vi "Multichannel Recording0.7.vi"() -> ()   [LabVIEW 2014]
uses:
  Multichannel Record/Enum State Typedef.ctl
  Consumer Data_ Consumer Event Com.ctl
  Multichannel Record/Data Producer States.ctl
  <vilib>/_DAQmxBase/Internals/DAQmxBase Read (Analog 2D DBL NChan NSamp).vi
  <vilib>/_DAQmxBase/Internals/DAQmxBase Create Channel (AI-Voltage-Basic).vi
  <vilib>/_DAQmxBase/Internals/DAQmxBase Timing (Sample Clock).vi
panel:
  out "Progress (% / 100)":dbl(slide) scale=0.0..1.0
  in  "Display Size":T1(ring)
  out "Total Iterations Needed":dbl
  out "Read Data":i32
  out "Data Producer State":T2=enum."Default"
  out "Data Consumer State":T3=enum."Default"
  in  "Open Button":bool
  in  "Tab Control":T4(tab)
  in  "Amplifier Channel 0":T5 {"Amplifier Model" items=["Select a Model", "AM 1700", "BMA 200"]}
  out "Channel 0 Chart":waveform(dbl)(graph)
  in  "User Data Channel 0":T6
  in  "Use Channel 0":bool caption="In Use?"
  out "Channel 1 Chart":waveform(dbl)(graph)
  in  "User Data Channel 1":T6
  in  "Amplifier Channel 1":T5 {"Amplifier Model" items=["Select a Model", "AM 1700", "BMA 200"]}
  in  "Use Channel 1":bool caption="In Use?"
  out "Channel 2 Chart":waveform(dbl)(graph)
  in  "User Data Channel 2":T6
  in  "Amplifier Channel 2":T5 {"Amplifier Model" items=["Select a Model", "AM 1700", "BMA 200"]}
  in  "Use Channel 2":bool caption="In Use?"
  out "Channel 3 Chart":waveform(dbl)(graph)
  in  "User Data Channel 3":T6
  in  "Amplifier Channel 3":T5 {"Amplifier Model" items=["Select a Model", "AM 1700", "BMA 200"]}
  in  "Use Channel 3":bool caption="In Use?"
  out "Overview Chart":waveform(dbl)[](graph)
  in  "Stop Preview":bool
  in  "OK Button":bool
  out "Event State":T7
  in  "Clear Display":bool
  in  "Preview Button":bool
  out "Iterations Recorded":i32
  in  "Recording Time (seconds)":dbl
  in  "Sample Rate":i64=1000
  in  "Stop Button":bool
  out "Start Time hr/min":string
  out "Date mm/dd/yy":string
  in  "Exit Button":bool
  in  "Record Button":bool
  # "MSU EFISH Lab Multi-Channel Electronic Pulse Recorder"
  # "Must enter numbers into here before you start"
  # "Blue for On\nOrange for Off"
  # "DC"
  # "AC"
  # "Blue for AC and Orange for DC"
  # "Blue for On\nOrange for Off"
  # "DC"
  # "AC"
  # "Blue for AC and Orange for DC"
  # "Blue for On\nOrange for Off"
  # "DC"
  # "AC"
  # "Blue for AC and Orange for DC"
  # "Blue for On\nOrange for Off"
  # "DC"
  # "AC"
  # "Blue for AC and Orange for DC"
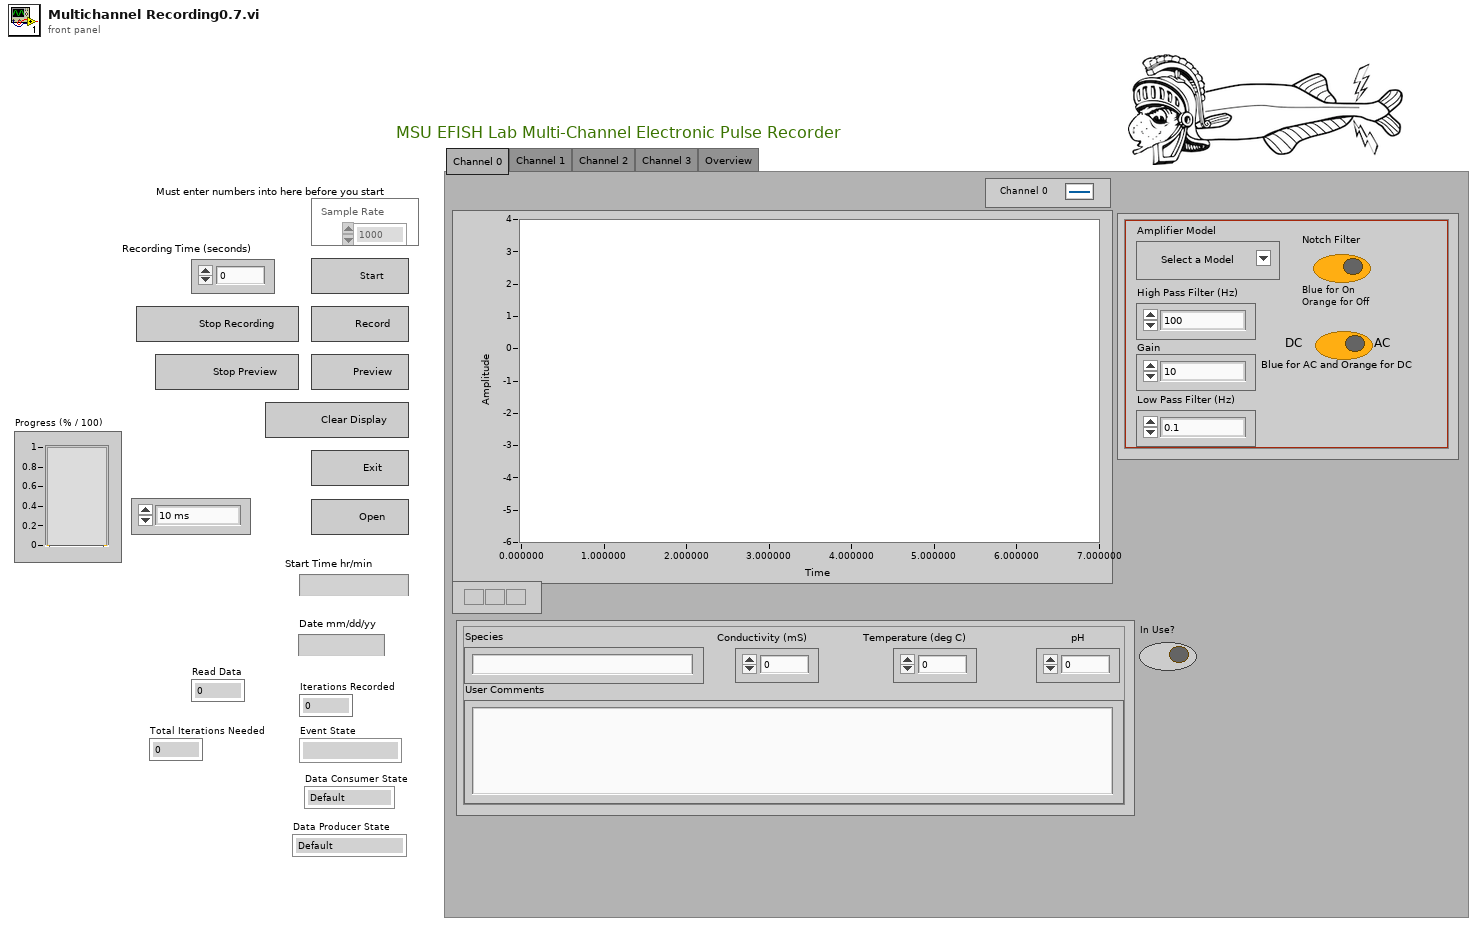
[diagram p1: front panel]
types:
  T1 = enum16{"10 ms", "100 ms", "1 Second", "10 sec", "30 sec"}
  T2 = typedef "Data Producer States.ctl" = enum16{"Read Data", "Set Sample Clock", "Default", "Exit", "Preview"}
  T3 = typedef "Consumer Data_ Consumer Event Com.ctl" = enum16{"Recording", "Create File", "Clear Memory", "Default", "End File", "Exit", "Set Sample Clock", "Preview"}
  T4 = enum32{"Channel 0", "Channel 1", "Channel 2", "Channel 3", "Overview"}
  T5 = cluster{"Low Pass Filter (Hz)":enum16{"0.1", "1", "3", "10", "30", "100", "300"}, "Gain ":enum16{"10", "20", "50", "100", "200", "500", "1000", "2k", "5k", "10k", "20k", "50k"}, "High Pass Filter (Hz)":enum16{"100", "500", "1000", "3000", "5000", "10,000", "20,000", "30,000", "50,000"}, "Notch Filter":bool, "Amplifier Model":u16, "AC/DC Switch":bool}
  T6 = cluster{"pH":dbl, "Conductivity (mS)":dbl, "Temperature (deg C)":dbl, "User Comments":string, "Species":string}
  T7 = typedef "Enum State Typedef.ctl" = enum16{"", "Open FIle", "Beginning State", "Set the Sample Clock", "Prepreview Handling", "Clear Display", "Preview Data", "Stop", "Exit", "Record", "Create File"}
  T8 = enum8{"Enabled", "Disabled", "Disabled and Grayed Out"}
  T9 = enum16{"Recording", "Create File", "Clear Memory", "Default"}
  T10 = cluster{"Refnum out":refnum<k34>, "Refnum out":refnum<k34>, "Refnum out":refnum<k34>, "Refnum out":refnum<k34>}
  T11 = cluster{"Use Channel 0":bool, "Use Channel 1":bool, "Use Channel 2":bool, "Use Channel 3":bool}
  T12 = cluster{"tdms file out":refnum<k34>, "tdms file out":refnum<k34>, "tdms file out":refnum<k34>, "tdms file out":refnum<k34>}
  T13 = cluster{"Channel 0 Chart":refnum<vi>, "Channel 1 Chart":refnum<vi>, "Channel 2 Chart":refnum<vi>, "Channel 3 Chart":refnum<vi>, "Overview Chart":refnum<vi>}
  T14 = cluster{"Waveform":waveform(dbl), "Waveform":waveform(dbl), "Waveform":waveform(dbl), "Waveform":waveform(dbl), waveform(dbl)[]}
  T15 = enum16{"Read Data", "Set Sample Clock", "Default", "Exit"}
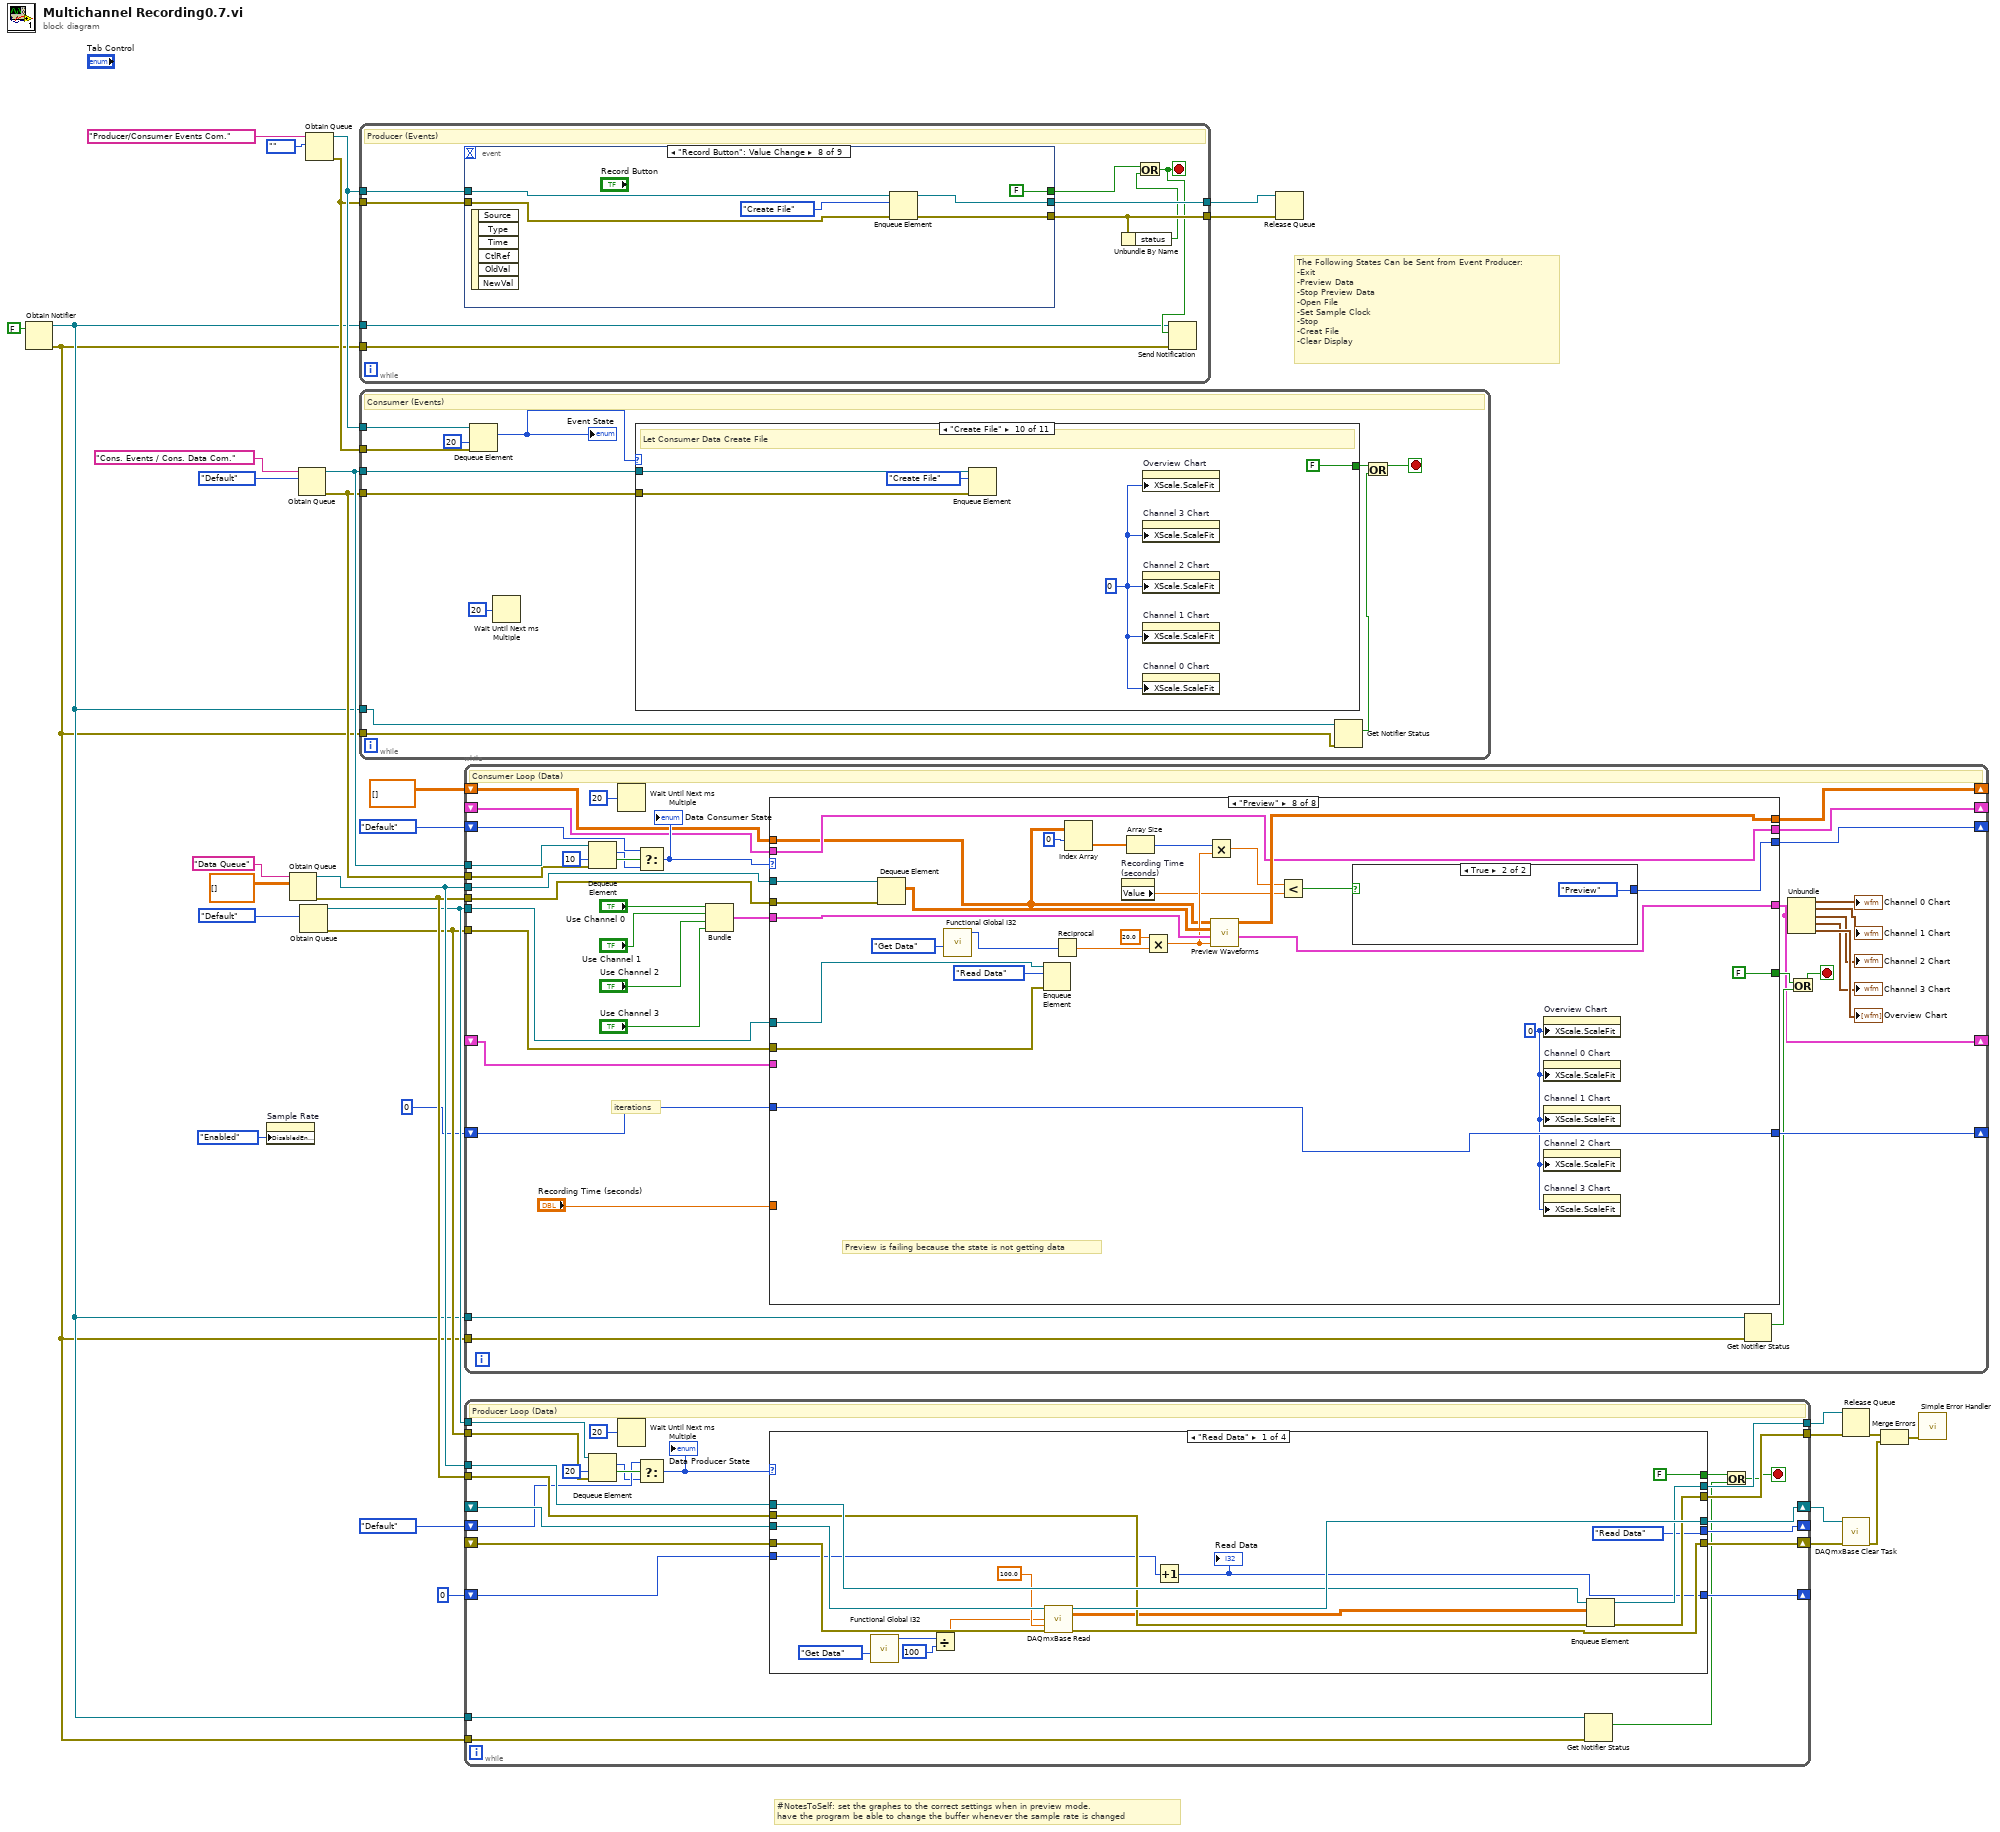
[diagram p0: block diagram]
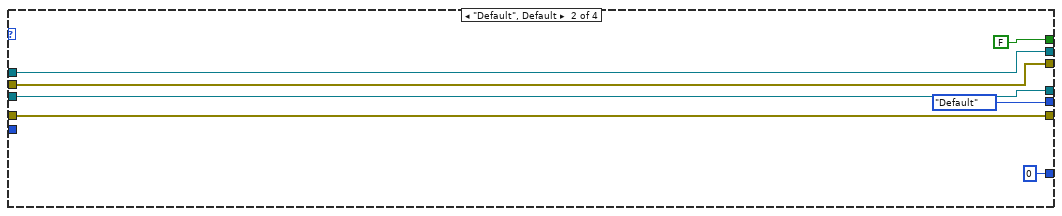
[diagram p2: hidden frame]
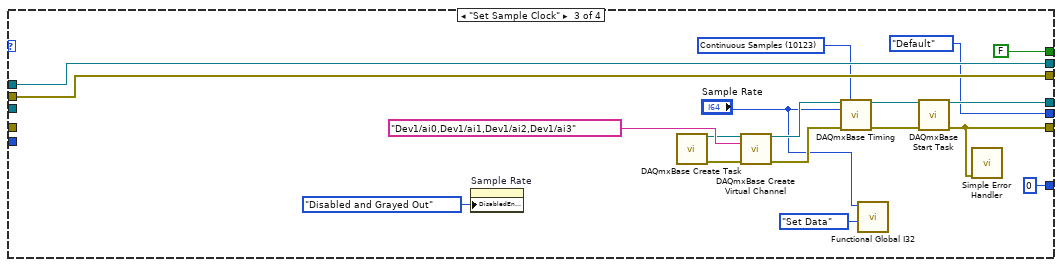
[diagram p3: hidden frame]
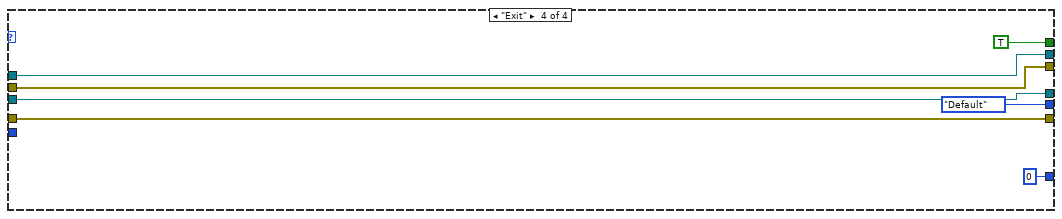
[diagram p4: hidden frame]
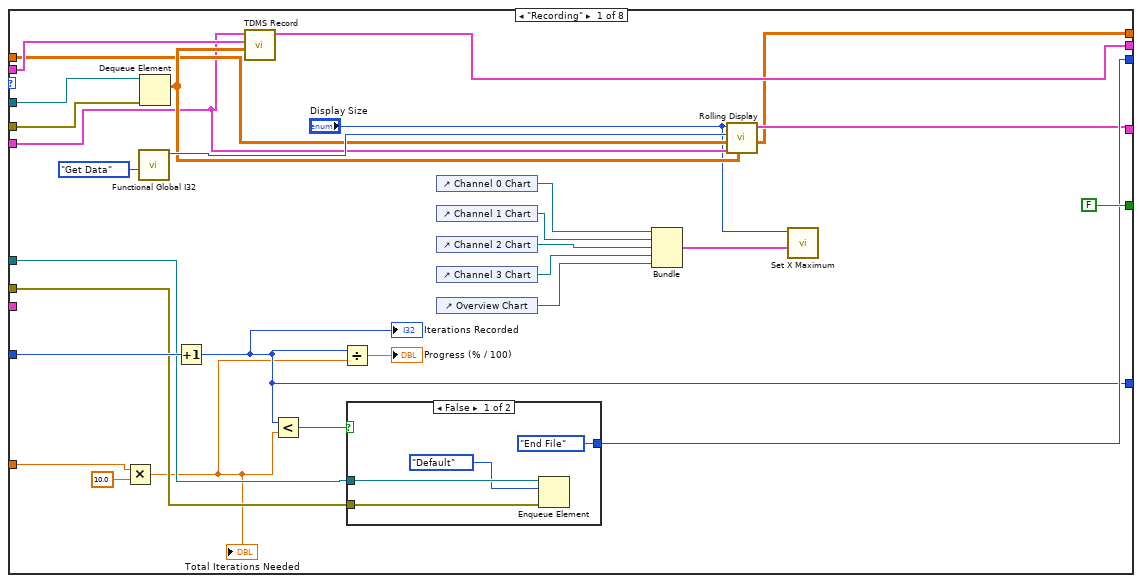
[diagram p5: hidden frame]
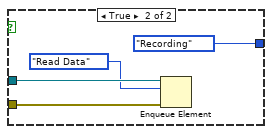
[diagram p6: hidden frame]
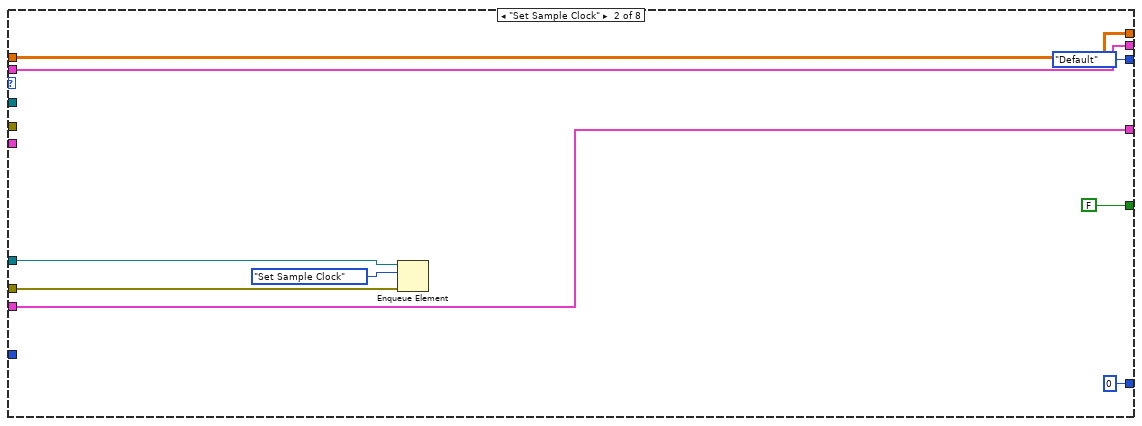
[diagram p7: hidden frame]
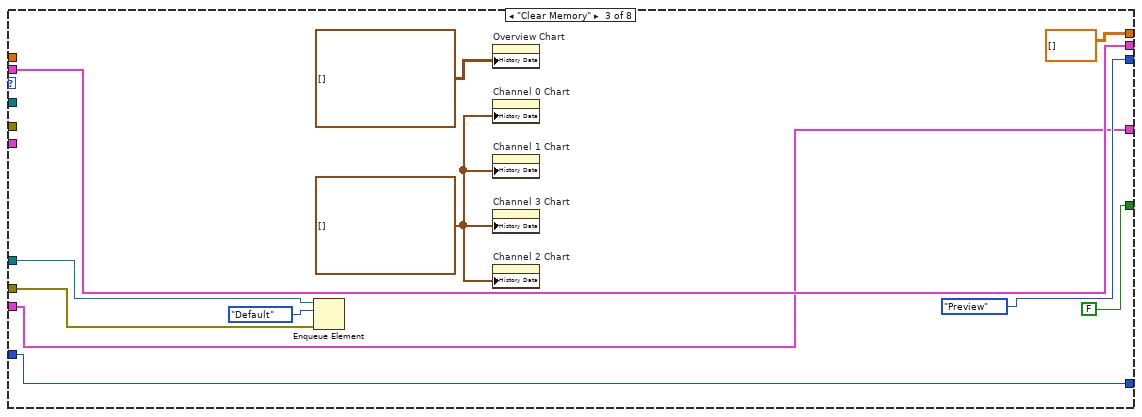
[diagram p8: hidden frame]
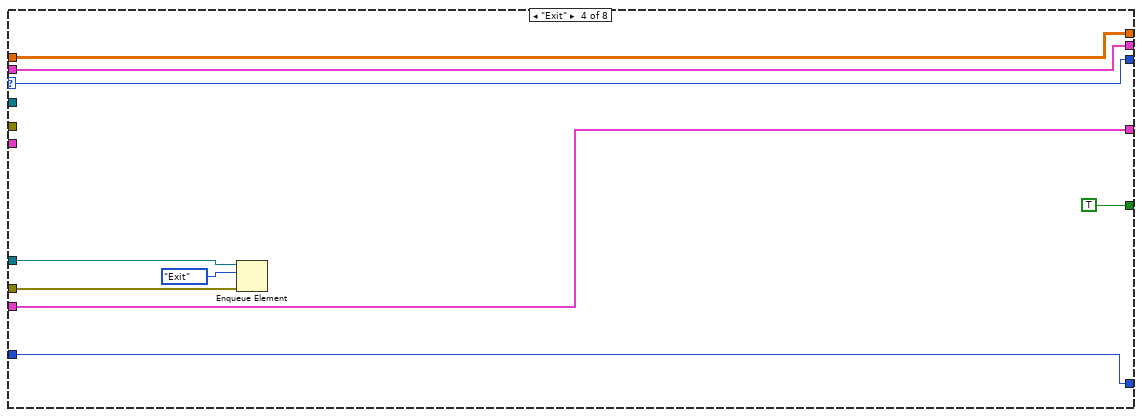
[diagram p9: hidden frame]
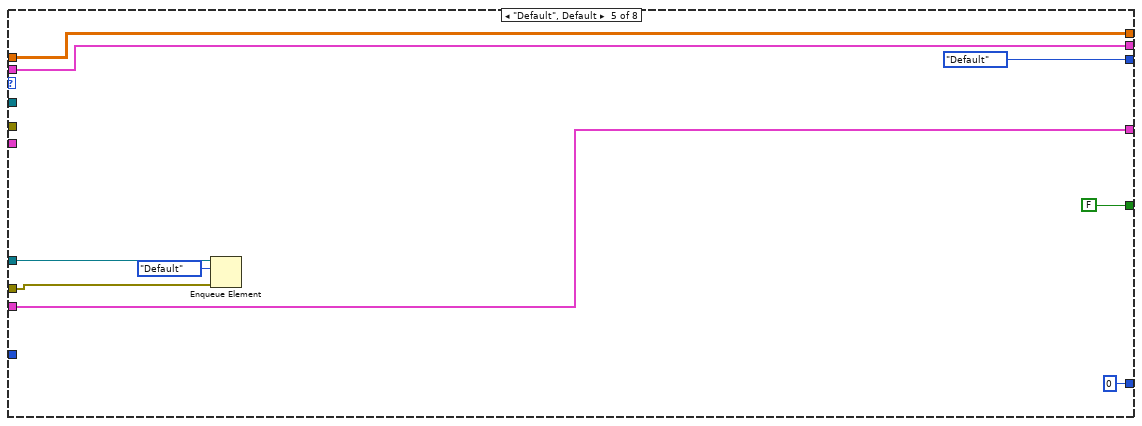
[diagram p10: hidden frame]
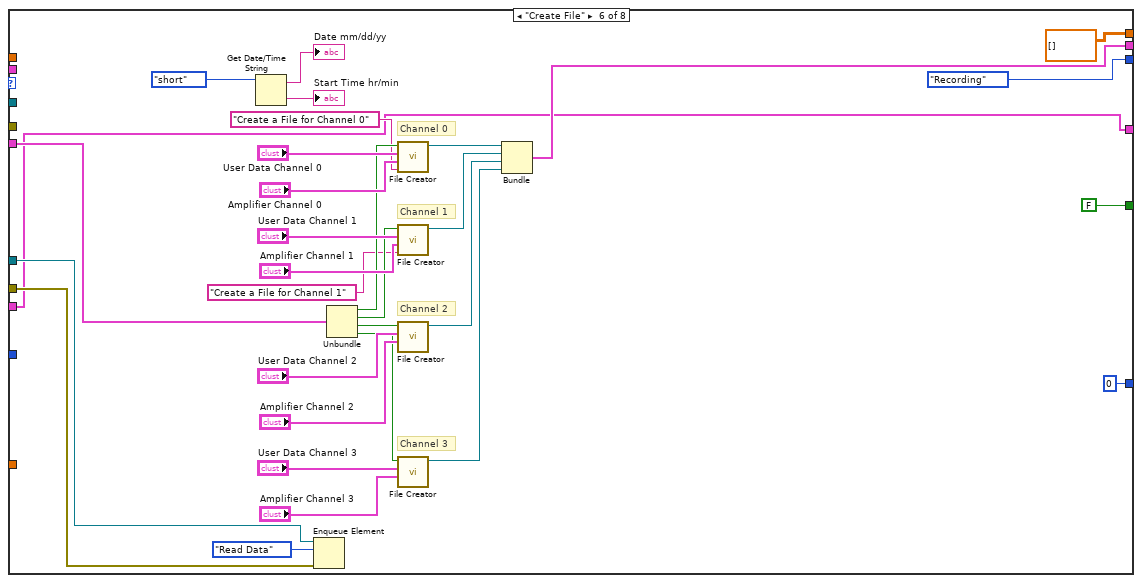
[diagram p11: hidden frame]
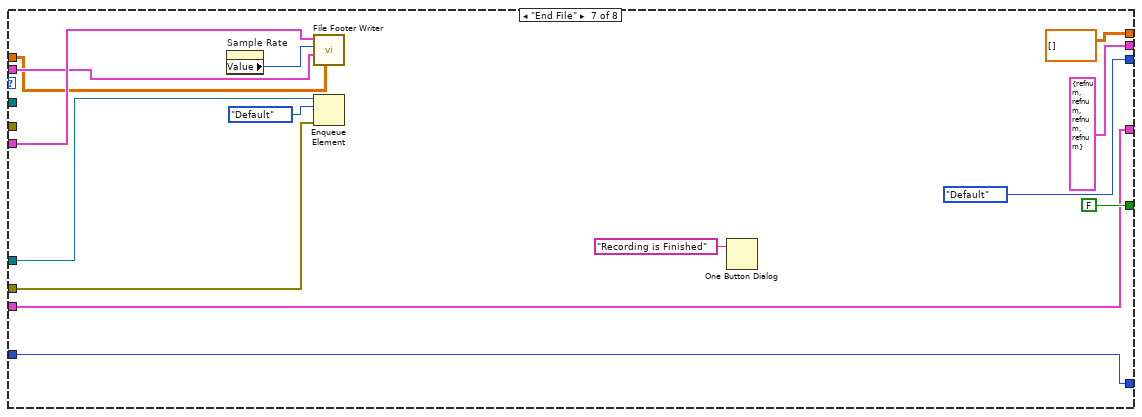
[diagram p12: hidden frame]
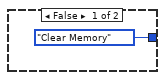
[diagram p13: hidden frame]
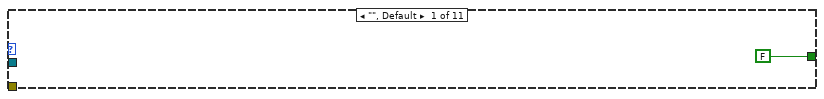
[diagram p14: hidden frame]
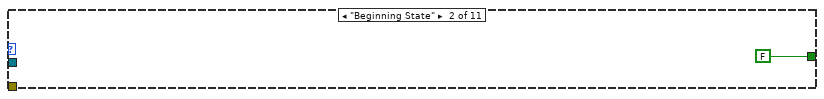
[diagram p15: hidden frame]
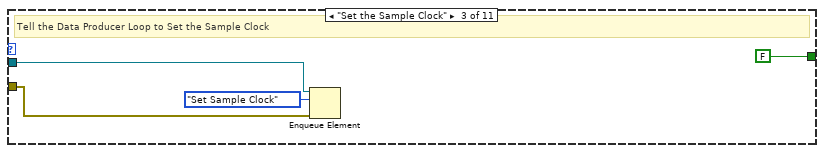
[diagram p16: hidden frame]
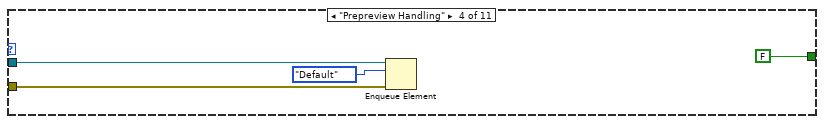
[diagram p17: hidden frame]
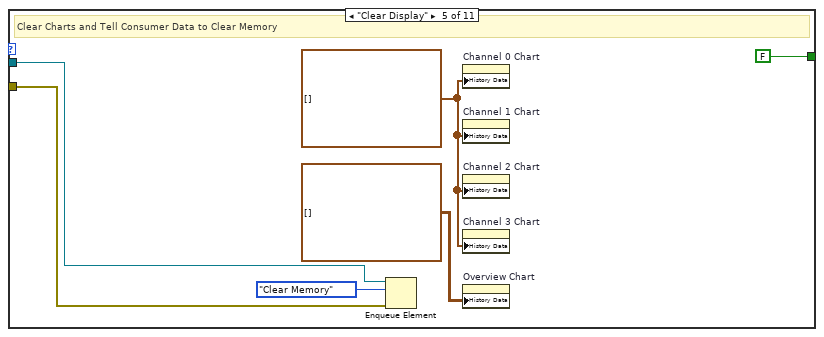
[diagram p18: hidden frame]
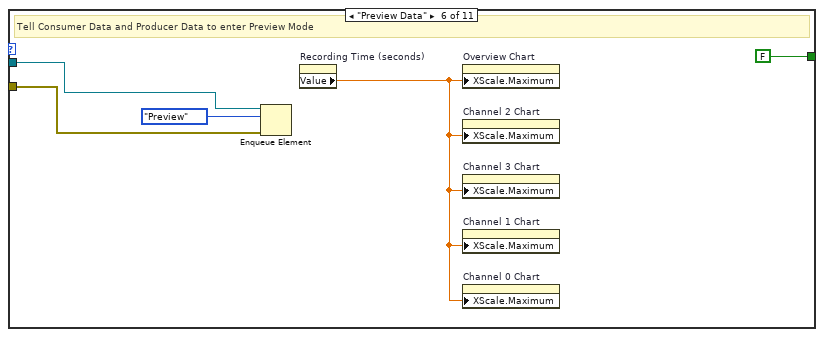
[diagram p19: hidden frame]
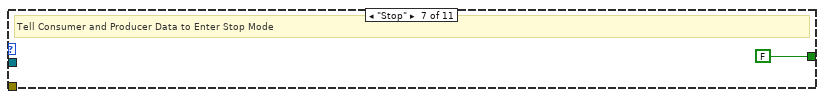
[diagram p20: hidden frame]
diagram:
  # "#NotesToSelf: set the graphes to the correct settings when in preview mode.\nhave the program be able to change the buffer whenever the sample rate is changed"
  # "The Following States Can be Sent from Event Producer:\n-Exit\n-Preview Data\n-Stop Preview Data\n-Open File\n-Set Sample Clock\n-Stop\n-Creat File\n-Clear Display"
  n1 = Obtain Notifier(notification data type=FALSE) -> (notifier out=w2:refnum<notifier>, error out=w1:errorcluster)  [unwired: 3 in, 1 out]
  n2 = property on="Sample Rate" class="DigNum (strict)"("DisabledEnum"=T8."Enabled" ("Disabled")) -> ()  [unwired: 2 in, 2 out]
  n3 = Obtain Queue(name (unnamed)="Data Queue", element data type=dbl[][] []) -> (queue out=w28:refnum<queue>, error out=w27:errorcluster)  [unwired: 3 in, 1 out]
  n4 = Obtain Queue(name (unnamed)="Cons. Events / Cons. Data Com.", element data type=Consumer_Data__Consumer_Event_Com."Default") -> (queue out=w20:refnum<queue>, error out=w19:errorcluster)  [unwired: 3 in, 1 out]
  n5 = Obtain Queue(element data type=Data_Producer_States."Default") -> (queue out=w9:refnum<queue>, error out=w8:errorcluster)  [unwired: 4 in, 1 out]
  n6 = Obtain Queue(name (unnamed)="Producer/Consumer Events Com.", element data type=Enum_State_Typedef."" ("State")) -> (queue out=w32:refnum<queue>, error out=w31:errorcluster)  [unwired: 3 in, 1 out]
  n7 = while {
    tunnel: w32 -> [w42]
    tunnel: w31 -> [w41]
    tunnel: [w40] -> w26
    tunnel: [w39] -> w25
    tunnel: w2 -> [w35]
    tunnel: w1 -> [w34]
    stop <- w36 stop-if-true
    # "Producer (Events)"
    n8 = event shown="[7] \"Record Button\": Value Change" {
      selector: _ -> [_ _ _ _ _ _ _ _ _]
      dyn-events: _ -> [_ _ _ _ _ _ _ _ _]
      timeout: _ -> [_ _ _ _ _ _ _ _ _]
      tunnel: [FALSE ("Exit Button") "Exit Button" FALSE ("Exit Button") FALSE ("Exit Button") FALSE ("Exit Button") FALSE ("Exit Button") FALSE ("Exit Button") FALSE ("Exit Button") FALSE ("Exit Button")] -> w38
      tunnel: w42 -> [w44 w50 w57 w63 w69 w75 w81 w87 w93]
      tunnel: w41 -> [w43 w49 w56 w62 w68 w74 w80 w86 w92]
      tunnel: [w44 w47 w53 w59 w65 w71 w77 w83 w89] -> w40
      tunnel: [w43 w46 w52 w58 w64 w70 w76 w82 w88] -> w39
      event Timeout {
        n9 = event-data() -> ()  [unwired: 1 in, 3 out]
      }
      event "Exit Button": Value Change {
        n10 = event-data() -> ()  [unwired: 1 in, 1 out]
        n11 = Enqueue Element(queue=w50, element=Enum_State_Typedef."Exit", error in (no error)=w49) -> (queue out=w47:refnum<queue>, error out=w46:errorcluster)  [unwired: 1 in, 1 out]
      }
      event "Preview Button": Value Change {
        n12 = event-data() -> ()  [unwired: 1 in, 6 out]
        n13 = Enqueue Element(queue=w57, element=Enum_State_Typedef."Preview Data", error in (no error)=w56) -> (queue out=w53:refnum<queue>, error out=w52:errorcluster)  [unwired: 1 in, 1 out]
      }
      event "Stop Preview": Value Change {
        n14 = event-data() -> ()  [unwired: 1 in, 6 out]
        n15 = Enqueue Element(queue=w63, element=Enum_State_Typedef."Prepreview Handling", error in (no error)=w62) -> (queue out=w59:refnum<queue>, error out=w58:errorcluster)  [unwired: 1 in, 1 out]
      }
      event "Open Button": Value Change {
        n16 = event-data() -> ()  [unwired: 1 in, 6 out]
        n17 = Enqueue Element(queue=w69, element=Enum_State_Typedef."Open FIle", error in (no error)=w68) -> (queue out=w65:refnum<queue>, error out=w64:errorcluster)  [unwired: 1 in, 1 out]
      }
      event "OK Button": Value Change {
        n18 = event-data() -> ()  [unwired: 1 in, 6 out]
        n19 = Enqueue Element(queue=w75, element=Enum_State_Typedef."Set the Sample Clock", error in (no error)=w74) -> (queue out=w71:refnum<queue>, error out=w70:errorcluster)  [unwired: 1 in, 1 out]
      }
      event "Stop Button": Value Change {
        n20 = event-data() -> ()  [unwired: 1 in, 6 out]
        n21 = Enqueue Element(queue=w81, element=Enum_State_Typedef."Stop", error in (no error)=w80) -> (queue out=w77:refnum<queue>, error out=w76:errorcluster)  [unwired: 1 in, 1 out]
      }
      event "Record Button": Value Change {
        n22 = event-data() -> ()  [unwired: 1 in, 6 out]
        n23 = Enqueue Element(queue=w87, element=Enum_State_Typedef."Create File", error in (no error)=w86) -> (queue out=w83:refnum<queue>, error out=w82:errorcluster)  [unwired: 1 in, 1 out]
      }
      event "Clear Display": Value Change {
        n24 = event-data() -> ()  [unwired: 1 in, 6 out]
        n25 = Enqueue Element(queue=w93, element=Enum_State_Typedef."Clear Display", error in (no error)=w92) -> (queue out=w89:refnum<queue>, error out=w88:errorcluster)  [unwired: 1 in, 1 out]
      }
    }
    n26 = Unbundle By Name(w39) -> ("status"=w37:bool)
    n27 = Or(x=w38, y=w37) -> (x .or. y?=w36:bool)
    n28 = Send Notification(notification=w36, notifier=w35, error in (no error)=w34) -> ()  [unwired: 2 out]
  }
  n29 = while {
    tunnel: w32 -> [w105]
    tunnel: w31 -> [w104]
    tunnel: w20 -> [w103]
    tunnel: w19 -> [w102]
    tunnel: w2 -> [w97]
    tunnel: w1 -> [w96]
    stop <- w95 stop-if-true
    # "Consumer (Events)"
    n30 = Dequeue Element(queue=w105, timeout in ms (-1)=20, error in (no error)=w104) -> (element=w100:T7)  [unwired: 3 out]
    "Event State" <- w100
    n31 = Wait Until Next ms Multiple(millisecond multiple=u32 20) -> ()  [unwired: 1 out]
    n32 = case shown="\"Create File\"" w100 {
      tunnel: w103 -> [_ _ w110 w114 w118 w124 _ w131 _ w136 _]
      tunnel: w102 -> [_ _ w109 w113 w117 w123 _ w130 _ w135 _]
      tunnel: [FALSE FALSE FALSE FALSE FALSE FALSE FALSE TRUE FALSE FALSE FALSE] -> w101
      frame "", Default {
      }
      frame "Beginning State" {
      }
      frame "Set the Sample Clock" {
        # "Tell the Data Producer Loop to Set the Sample Clock"
        n33 = Enqueue Element(queue=w110, element=Consumer_Data__Consumer_Event_Com."Set Sample Clock", error in (no error)=w109) -> ()  [unwired: 1 in, 3 out]
      }
      frame "Prepreview Handling" {
        n34 = Enqueue Element(queue=w114, element=Consumer_Data__Consumer_Event_Com."Default", error in (no error)=w113) -> ()  [unwired: 1 in, 3 out]
      }
      frame "Clear Display" {
        w120 = waveform(dbl)[] [] ("History Data")
        # "Clear Charts and Tell Consumer Data to Clear Memory"
        n35 = Enqueue Element(queue=w118, element=Consumer_Data__Consumer_Event_Com."Clear Memory", error in (no error)=w117) -> ()  [unwired: 1 in, 3 out]
        n36 = property on="Channel 0 Chart" class="WFChart (strict)"("History Data"=w120) -> ()  [unwired: 2 in, 2 out]
        n37 = property on="Channel 1 Chart" class="WFChart (strict)"("History Data"=w120) -> ()  [unwired: 2 in, 2 out]
        n38 = property on="Channel 2 Chart" class="WFChart (strict)"("History Data"=w120) -> ()  [unwired: 2 in, 2 out]
        n39 = property on="Channel 3 Chart" class="WFChart (strict)"("History Data"=w120) -> ()  [unwired: 2 in, 2 out]
        n40 = property on="Overview Chart" class="WFChart (strict)"("History Data"=waveform(dbl)[][] []) -> ()  [unwired: 2 in, 2 out]
      }
      frame "Preview Data" {
        # "Tell Consumer Data and Producer Data to enter Preview Mode"
        n41 = Enqueue Element(queue=w124, element=Consumer_Data__Consumer_Event_Com."Preview", error in (no error)=w123) -> ()  [unwired: 1 in, 3 out]
        n42 = property on="Recording Time (seconds)" class="DigNum (strict)"() -> ("Value"=w125:dbl)  [unwired: 2 in, 2 out]
        n43 = property on="Overview Chart" class="WFChart (strict)"("XScale.Maximum"=w125) -> ()  [unwired: 2 in, 2 out]
        n44 = property on="Channel 2 Chart" class="WFChart (strict)"("XScale.Maximum"=w125) -> ()  [unwired: 2 in, 2 out]
        n45 = property on="Channel 3 Chart" class="WFChart (strict)"("XScale.Maximum"=w125) -> ()  [unwired: 2 in, 2 out]
        n46 = property on="Channel 1 Chart" class="WFChart (strict)"("XScale.Maximum"=w125) -> ()  [unwired: 2 in, 2 out]
        n47 = property on="Channel 0 Chart" class="WFChart (strict)"("XScale.Maximum"=w125) -> ()  [unwired: 2 in, 2 out]
      }
      frame "Stop" {
        # "Tell Consumer and Producer Data to Enter Stop Mode"
      }
      frame "Exit" {
        # "Tell Producer and Consumer Data to end themselves then End the Program"
        n48 = Enqueue Element(queue=w131, element=Consumer_Data__Consumer_Event_Com."Exit", error in (no error)=w130) -> ()  [unwired: 1 in, 3 out]
      }
      frame "Record" {
        # "(I dont think that this case will exist)"
      }
      frame "Create File" {
        w133 = u8 0 ("X Scale.Scale Fit")
        # "Let Consumer Data Create File"
        n49 = Enqueue Element(queue=w136, element=Consumer_Data__Consumer_Event_Com."Create File", error in (no error)=w135) -> ()  [unwired: 1 in, 3 out]
        n50 = property on="Overview Chart" class="WFChart (strict)"("XScale.ScaleFit"=w133) -> ()  [unwired: 2 in, 2 out]
        n51 = property on="Channel 3 Chart" class="WFChart (strict)"("XScale.ScaleFit"=w133) -> ()  [unwired: 2 in, 2 out]
        n52 = property on="Channel 2 Chart" class="WFChart (strict)"("XScale.ScaleFit"=w133) -> ()  [unwired: 2 in, 2 out]
        n53 = property on="Channel 1 Chart" class="WFChart (strict)"("XScale.ScaleFit"=w133) -> ()  [unwired: 2 in, 2 out]
        n54 = property on="Channel 0 Chart" class="WFChart (strict)"("XScale.ScaleFit"=w133) -> ()  [unwired: 2 in, 2 out]
      }
      frame "Open FIle" {
        # "Tell the Data Consumer to Create the File"
        n55 = call "File Dialog"() -> ("selected path"=w138:path)  [unwired: 12 in, 3 out]
        n56 = call <vilib>:"TDMS - File Viewer.vi"("file path"=w138) -> ()  [unwired: 5 in, 2 out]
      }
    }
    n57 = Get Notifier Status(notifier=w97, error in (no error)=w96) -> (current notification=w94:bool)  [unwired: 4 out]
    n58 = Or(x=w101, y=w94) -> (x .or. y?=w95:bool)
  }
  n59 = while {
    tunnel: w28 -> [w169]
    tunnel: w27 -> [w168]
    tunnel: w20 -> [w176]
    tunnel: w19 -> [w175]
    shift-right: [w170] -> _
    shift-left: Consumer_Data__Consumer_Event_Com."Default" -> [w171]
    shift-right: [w164] -> _
    shift-left: dbl[][] [] -> [w167]
    shift-right: [w163] -> _
    shift-left: _ -> [w162]
    tunnel: w9 -> [w160]
    tunnel: w8 -> [w159]
    shift-right: [w155] -> _
    shift-left: 0 -> [w157]
    tunnel: w2 -> [w149]
    tunnel: w1 -> [w148]
    shift-right: [w141] -> _
    shift-left: _ -> [w140]
    stop <- w151 stop-if-true
    # "iterations"
    # "Consumer Loop (Data)"
    n60 = Dequeue Element(queue=w176, timeout in ms (-1)=10, error in (no error)=w175) -> (element=w173:T3, timed out?=w174:bool)  [unwired: 2 out]
    n61 = Wait Until Next ms Multiple(millisecond multiple=u32 20) -> ()  [unwired: 1 out]
    n62 = Select(t=w171, s=w174, f=w173) -> (s? t:f=w172:T3)
    "Data Consumer State" <- w172
    n63 = Bundle("Use Channel 0"="Use Channel 0", "Use Channel 1"="Use Channel 1", "Use Channel 2"="Use Channel 2", "Use Channel 3"="Use Channel 3") -> (w165:T11)  [unwired: 1 in]
    n64 = case shown="\"Preview\"" w172 {
      selector: w172 -> [_ _ _ w240 _ _ _ _]
      tunnel: [w197 Consumer_Data__Consumer_Event_Com."Default" Consumer_Data__Consumer_Event_Com."Preview" w240 T9."Default" Consumer_Data__Consumer_Event_Com."Recording" Consumer_Data__Consumer_Event_Com."Default" w306] -> w170
      tunnel: w169 -> [w204 _ _ _ _ _ _ w322]
      tunnel: w168 -> [w203 _ _ _ _ _ _ w321]
      tunnel: [FALSE FALSE FALSE TRUE FALSE FALSE FALSE FALSE] -> w150
      tunnel: w167 -> [w190 w219 _ w241 w249 _ w294 w313]
      tunnel: w165 -> [w189 _ _ _ _ w276 w296 w319]
      tunnel: [w187 w219 dbl[][] [] ("Output Decimated Data") w241 w249 dbl[][] [] ("Output Decimated Data") dbl[][] [] ("Output Data") w316] -> w164
      tunnel: [w202 w218 w230 w239 w248 w259 T10 {"Refnum out"=refnum, "Refnum out"=refnum, "Refnum out"=refnum, "Refnum out"=refnum} ("Output TDMS File Cluster") w315] -> w163
      tunnel: w162 -> [w194 w218 w230 w239 w248 _ w295 w315]
      tunnel: w160 -> [w196 w222 w227 w238 w246 w258 w288 w304]
      tunnel: w159 -> [w195 w221 w226 w237 w245 w257 w287 w303]
      tunnel: w157 -> [w201 _ w224 w235 _ _ w285 w301]
      tunnel: "Recording Time (seconds)" -> [w200 _ _ _ _ _ _ _]
      tunnel: [w179 0 w224 w235 0 0 w285 w301] -> w155
      tunnel: [w188 w214 w223 w234 w243 w252 w283 w297] -> w141
      tunnel: w140 -> [_ w214 w223 w234 w243 w252 w283 _]
      frame "Recording" {
        n65 = Multiply(x=w200, y=10.0) -> (x*y=w178:dbl)
        "Total Iterations Needed" <- w178
        n66 = call "Functional Global I32.vi"("Enum"=enum16{"Set Data", "Get Data"}."Get Data") -> ("Integer"=w192:i32)  [unwired: 10 in]
        n67 = Dequeue Element(queue=w204, error in (no error)=w203) -> (element=w191:dbl[][])  [unwired: 1 in, 3 out]
        n68 = Increment(x=w201) -> (x+1=w179:i32)
        "Iterations Recorded" <- w179
        n69 = call "TDMS Record.vi"("Data"=w191, "Input TDMS File Cluster"=w194, "In Use Cluster"=w189) -> ("Output TDMS File Cluster"=w202:T12)  [unwired: 8 in]
        n70 = Less?(x=w179, y=w178) -> (x < y?=w198:bool)
        n71 = Divide(x=w179, y=w178) -> (x/y=→"Progress (% / 100)":dbl)
        n72 = case shown="False" w198 {
          tunnel: [Consumer_Data__Consumer_Event_Com."End File" Consumer_Data__Consumer_Event_Com."Recording"] -> w197
          tunnel: w196 -> [w208 w212]
          tunnel: w195 -> [w207 w211]
          frame False {
            n73 = Enqueue Element(queue=w208, element=Data_Producer_States."Default", error in (no error)=w207) -> ()  [unwired: 1 in, 3 out]
          }
          frame True {
            n74 = Enqueue Element(queue=w212, element=Data_Producer_States."Read Data", error in (no error)=w211) -> ()  [unwired: 1 in, 3 out]
          }
        }
        n75 = control-ref of="Channel 0 Chart"() -> (w186:refnum<vi>)
        n76 = control-ref of="Channel 1 Chart"() -> (w185:refnum<vi>)
        n77 = control-ref of="Channel 2 Chart"() -> (w184:refnum<vi>)
        n78 = control-ref of="Channel 3 Chart"() -> (w183:refnum<vi>)
        n79 = control-ref of="Overview Chart"() -> (w182:refnum<vi>)
        n80 = Bundle("Channel 0 Chart"=w186, "Channel 1 Chart"=w185, "Channel 2 Chart"=w184, "Channel 3 Chart"=w183, "Overview Chart"=w182) -> (w181:T13)  [unwired: 1 in]
        n81 = call "Rolling Display.vi"("Input Data"=w191, "Channels in Use"=w189, "Old Data"=w190, "Sample Rate"=w192, "Display Size"="Display Size") -> ("Output Array Values"=w187:dbl[][], "Output Waveform Cluster"=w188:T14)  [unwired: 5 in]
        n82 = call "Set X Maximum.vi"("Waveform Reference Cluster"=w181, "Display Size"="Display Size") -> ()  [unwired: 10 in]
      }
      frame "Set Sample Clock" {
        n83 = Enqueue Element(queue=w222, element=Data_Producer_States."Set Sample Clock", error in (no error)=w221) -> ()  [unwired: 1 in, 3 out]
      }
      frame "Clear Memory" {
        w228 = waveform(dbl)[] [] ("History Data")
        n84 = Enqueue Element(queue=w227, element=Data_Producer_States."Default", error in (no error)=w226) -> ()  [unwired: 1 in, 3 out]
        n85 = property on="Overview Chart" class="WFChart (strict)"("History Data"=waveform(dbl)[][] []) -> ()  [unwired: 2 in, 2 out]
        n86 = property on="Channel 0 Chart" class="WFChart (strict)"("History Data"=w228) -> ()  [unwired: 2 in, 2 out]
        n87 = property on="Channel 1 Chart" class="WFChart (strict)"("History Data"=w228) -> ()  [unwired: 2 in, 2 out]
        n88 = property on="Channel 3 Chart" class="WFChart (strict)"("History Data"=w228) -> ()  [unwired: 2 in, 2 out]
        n89 = property on="Channel 2 Chart" class="WFChart (strict)"("History Data"=w228) -> ()  [unwired: 2 in, 2 out]
      }
      frame "Exit" {
        n90 = Enqueue Element(queue=w238, element=Data_Producer_States."Exit", error in (no error)=w237) -> ()  [unwired: 1 in, 3 out]
      }
      frame "Default", Default {
        n91 = Enqueue Element(queue=w246, element=Data_Producer_States."Default", error in (no error)=w245) -> ()  [unwired: 1 in, 3 out]
      }
      frame "Create File" {
        # "Channel 3"
        # "Channel 2"
        # "Channel 1"
        # "Channel 0"
        n92 = Get Date/Time String(date format (0)=enum16{"short", "long", "abbreviated"}."short") -> (date string=→"Date mm/dd/yy":string, time string=→"Start Time hr/min":string)  [unwired: 2 in]
        n93 = Enqueue Element(queue=w258, element=Data_Producer_States."Read Data", error in (no error)=w257) -> ()  [unwired: 1 in, 3 out]
        n94 = Unbundle(w276) -> ("Use Channel 0"=w269:bool, "Use Channel 1"=w268:bool, "Use Channel 2"=w267:bool, "Use Channel 3"=w266:bool)
        n95 = call "File Creator.vi"("prompt"="Create a File for Channel 0", "Amplifier Channel 1"="Amplifier Channel 0", "User Data Channel 1"="User Data Channel 0", "Use Channel in"=w269) -> ("Refnum out"=w265:refnum<k34>)  [unwired: 7 in]
        n96 = call "File Creator.vi"("prompt"="Create a File for Channel 1", "Amplifier Channel 1"="Amplifier Channel 1", "User Data Channel 1"="User Data Channel 1", "Use Channel in"=w268) -> ("Refnum out"=w264:refnum<k34>)  [unwired: 7 in]
        n97 = call "File Creator.vi"("Amplifier Channel 1"="Amplifier Channel 2", "User Data Channel 1"="User Data Channel 2", "Use Channel in"=w267) -> ("Refnum out"=w263:refnum<k34>)  [unwired: 8 in]
        n98 = call "File Creator.vi"("Amplifier Channel 1"="Amplifier Channel 3", "User Data Channel 1"="User Data Channel 3", "Use Channel in"=w266) -> ("Refnum out"=w262:refnum<k34>)  [unwired: 8 in]
        n99 = Bundle("Refnum out"=w265, "Refnum out"=w264, "Refnum out"=w263, "Refnum out"=w262) -> (w259:T10)  [unwired: 1 in]
      }
      frame "End File" {
        n100 = property on="Sample Rate" class="DigNum (strict)"() -> ("Value"=w293:i64)  [unwired: 2 in, 2 out]
        n101 = call "File Footer Writer.vi"("Old Data"=w294, "TDMS File Cluster"=w295, "Sample Rate"=w293, "In Use Cluster"=w296) -> ()  [unwired: 8 in]
        n102 = Enqueue Element(queue=w288, element=Data_Producer_States."Default", error in (no error)=w287) -> ()  [unwired: 1 in, 3 out]
        n103 = One Button Dialog(message="Recording is Finished") -> ()  [unwired: 1 in, 1 out]
      }
      frame "Preview" {
        w298 = u8 0 ("X Scale.Scale Fit")
        # "Preview is failing because the state is not getting data"
        n104 = Dequeue Element(queue=w322, error in (no error)=w321) -> (element=w320:dbl[][])  [unwired: 1 in, 3 out]
        n105 = call "Functional Global I32.vi"("Enum"=enum16{"Set Data", "Get Data"}."Get Data") -> ("Integer"=w299:i32)  [unwired: 10 in]
        n106 = Enqueue Element(queue=w304, element=Data_Producer_States."Read Data", error in (no error)=w303) -> ()  [unwired: 1 in, 3 out]
        n107 = Reciprocal(x=w299) -> (1/x=w318:dbl)
        n108 = Index Array(array=w313, index (row)=0) -> (element=w311:dbl[])  [unwired: 1 in]
        n109 = property on="Recording Time (seconds)" class="DigNum (strict)"() -> ("Value"=w308:dbl)  [unwired: 2 in, 2 out]
        n110 = Array Size(array=w311) -> (size(s)=w310:i32)
        n111 = Multiply(x=20.0, y=w318) -> (x*y=w314:dbl)
        n112 = Multiply(x=w310, y=w314) -> (x*y=w309:dbl)
        n113 = call "Preview Waveforms.vi"("Change in Time"=w314, "In Use Cluster"=w319, "Input Read Data"=w320, "Input Decimated Data"=w313) -> ("Output Waveform Cluster"=w297:T14, "Output Data"=w316:dbl[][])  [unwired: 6 in]
        n114 = Less?(x=w309, y=w308) -> (x < y?=w307:bool)
        n115 = case shown="True" w307 {
          tunnel: [Consumer_Data__Consumer_Event_Com."Clear Memory" Consumer_Data__Consumer_Event_Com."Preview"] -> w306
          frame False {
          }
          frame True {
          }
        }
        n116 = property on="Overview Chart" class="WFChart (strict)"("XScale.ScaleFit"=w298) -> ()  [unwired: 2 in, 2 out]
        n117 = property on="Channel 0 Chart" class="WFChart (strict)"("XScale.ScaleFit"=w298) -> ()  [unwired: 2 in, 2 out]
        n118 = property on="Channel 1 Chart" class="WFChart (strict)"("XScale.ScaleFit"=w298) -> ()  [unwired: 2 in, 2 out]
        n119 = property on="Channel 2 Chart" class="WFChart (strict)"("XScale.ScaleFit"=w298) -> ()  [unwired: 2 in, 2 out]
        n120 = property on="Channel 3 Chart" class="WFChart (strict)"("XScale.ScaleFit"=w298) -> ()  [unwired: 2 in, 2 out]
      }
    }
    n121 = Get Notifier Status(notifier=w149, error in (no error)=w148) -> (current notification=w147:bool)  [unwired: 4 out]
    n122 = Unbundle(w141) -> ("Waveform"=→"Channel 0 Chart":waveform(dbl), "Waveform"=→"Channel 1 Chart":waveform(dbl), "Waveform"=→"Channel 2 Chart":waveform(dbl), "Waveform"=→"Channel 3 Chart":waveform(dbl), →"Overview Chart":waveform(dbl)[])
    n123 = Or(x=w150, y=w147) -> (x .or. y?=w151:bool)
  }
  n124 = while {
    tunnel: w28 -> [w348]
    tunnel: w27 -> [w345]
    tunnel: [w347] -> w24
    tunnel: [w346] -> w23
    shift-right: [w333] -> _
    shift-left: Data_Producer_States."Default" -> [w326]
    shift-right: [w344] -> w17
    shift-left: _ -> [w342]
    shift-right: [w343] -> w16
    shift-left: _ -> [w341]
    tunnel: w9 -> [w338]
    tunnel: w8 -> [w337]
    shift-right: [w331] -> _
    shift-left: 0 -> [w332]
    tunnel: w2 -> [w328]
    tunnel: w1 -> [w327]
    stop <- w330 stop-if-true
    # "Producer Loop (Data)"
    n125 = Dequeue Element(queue=w338, timeout in ms (-1)=20, error in (no error)=w337) -> (element=w325:T2, timed out?=w336:bool)  [unwired: 2 out]
    n126 = Wait Until Next ms Multiple(millisecond multiple=u32 20) -> ()  [unwired: 1 out]
    n127 = Select(t=w326, s=w336, f=w325) -> (s? t:f=w335:T2)
    "Data Producer State" <- w335
    n128 = case shown="\"Read Data\"" w335 {
      tunnel: w348 -> [w362 w373 w383 w394]
      tunnel: [w360 w373 w383 w394] -> w347
      tunnel: [w359 w372 w382 w395] -> w346
      tunnel: w345 -> [w361 w372 w382 w395]
      tunnel: [w364 w371 w384 w396] -> w344
      tunnel: [w363 w370 w374 w397] -> w343
      tunnel: w342 -> [w366 w371 _ w396]
      tunnel: w341 -> [w365 w370 _ w397]
      tunnel: [FALSE FALSE FALSE TRUE] -> w339
      tunnel: [Data_Producer_States."Read Data" Data_Producer_States."Default" T15."Default" Data_Producer_States."Default"] -> w333
      tunnel: w332 -> [w355 _ _ _]
      tunnel: [w354 0 0 0] -> w331
      frame "Read Data" {
        n129 = call "Functional Global I32.vi"("Enum"=enum16{"Set Data", "Get Data"}."Get Data") -> ("Integer"=w351:i32)  [unwired: 10 in]
        n130 = Divide(x=w351, y=100) -> (x/y=w350:dbl)
        n131 = call-poly <vilib>:"DAQmxBase Read.vi"("task/channels in"=w366, "number of samples per channel"=w350, "timeout"=100.0, "error in"=w365) -> ("task out"=w364:refnum<k21>, "data"=w349:dbl[][], "error out"=w363:errorcluster)  [unwired: 9 in]
        n132 = Increment(x=w355) -> (x+1=w354:i32)
        "Read Data" <- w354
        n133 = Enqueue Element(queue=w362, element=w349, error in (no error)=w361) -> (queue out=w360:refnum<queue>, error out=w359:errorcluster)  [unwired: 1 in, 1 out]
      }
      frame "Default", Default {
      }
      frame "Set Sample Clock" {
        w375 = 10123 items=["Finite Samples"=10178, "Continuous Samples"=10123, "Hardware Timed Single Point"=12522] ("sample mode")
        n134 = property on="Sample Rate" class="DigNum (strict)"("DisabledEnum"=T8."Disabled and Grayed Out" ("Disabled")) -> ()  [unwired: 2 in, 2 out]
        n135 = call <vilib>:"DAQmxBase Create Task.vi"() -> ("task out"=w390:refnum<k21>, "error out"=w389:errorcluster)  [unwired: 14 in]
        n136 = call-poly <vilib>:"DAQmxBase Create Virtual Channel.vi"("task in"=w390, "physical channels"=tag "Dev1/ai0,Dev1/ai1,Dev1/ai2,Dev1/ai3", "error in"=w389) -> ("task out"=w387:refnum<k21>, "error out"=w388:errorcluster)  [unwired: 11 in]
        n137 = call-poly <vilib>:"DAQmxBase Timing.vi"("task/channels in"=w387, "sample mode"=w375, "rate"="Sample Rate", "error in"=w388) -> ("task out"=w386:refnum<k21>, "error out"=w385:errorcluster)  [unwired: 10 in]
        n138 = call "Functional Global I32.vi"("Enum"=enum16{"Set Data", "Get Data"}."Set Data", "Integer In"="Sample Rate") -> ()  [unwired: 9 in, 1 out]
        n139 = call <vilib>:"DAQmxBase Start Task.vi"("task/channels in"=w386, "error in"=w385) -> ("task out"=w384:refnum<k21>, "error out"=w374:errorcluster)  [unwired: 12 in]
        n140 = call <vilib>:"Simple Error Handler.vi"("error in (no error)"=w374) -> ()  [unwired: 4 in, 5 out]
      }
      frame "Exit" {
      }
    }
    n141 = Get Notifier Status(notifier=w328, error in (no error)=w327) -> (current notification=w329:bool)  [unwired: 4 out]
    n142 = Or(x=w339, y=w329) -> (x .or. y?=w330:bool)
  }
  n143 = Release Queue(queue=w26, error in (no error)=w25) -> ()  [unwired: 1 in, 3 out]
  n144 = Release Queue(queue=w24, error in (no error)=w23) -> (error out=w15:errorcluster)  [unwired: 1 in, 2 out]
  n145 = call <vilib>:"DAQmxBase Clear Task.vi"("task in"=w17, "error in"=w16) -> ("error out"=w14:errorcluster)  [unwired: 13 in]
  n146 = Merge Errors(w15, w14) -> (w13:errorcluster)
  n147 = call <vilib>:"Simple Error Handler.vi"("error in (no error)"=w13) -> ()  [unwired: 4 in, 5 out]
